vi "DTACQ - Read Data Size per Sample.vi"(8 "error in":errorcluster, 11 "Address":string) -> (0 "error out":errorcluster, 2 "Data Size":T1)   [LabVIEW 2017, in "Communications Library.lvlib"]
doc: "Read the size of data, for each sample point, from the analog in module. (eg. 16 bit or 32 bit dats?)"
uses:
  Communications Library.lvlib
  Typedefs/Data Size--Enum.ctl
  Typedefs/DTACQ Device Type--Enum.ctl
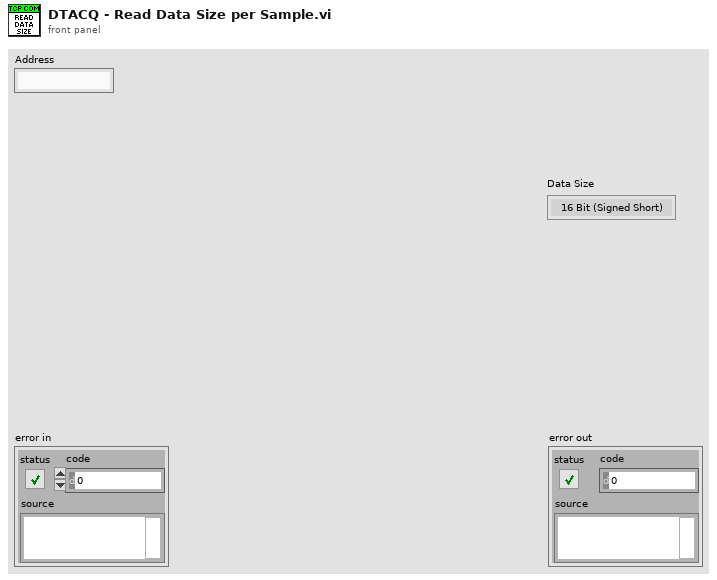
[diagram p1: front panel]
types:
  T1 = typedef "Communications Library.lvlib/Data Size--Enum.ctl" = enum16{"16 Bit (Signed Short)", "32 Bit (Signed Long)"}
  T2 = typedef "Communications Library.lvlib/DTACQ Device Type--Enum.ctl" = enum16{"Carrier", "Analog In Module", "Analog Out Module", "Generic Module"}
  T3 = typedef "Communications Library.lvlib/DTACQ Connection Data--Cluster.ctl" = cluster{"Description":string, "Address":string, "Port":u16, "timeout (ms)":i32, "Termination Character":string, "TCP Connection Reference":refnum<k5>, "Open Connection":bool}
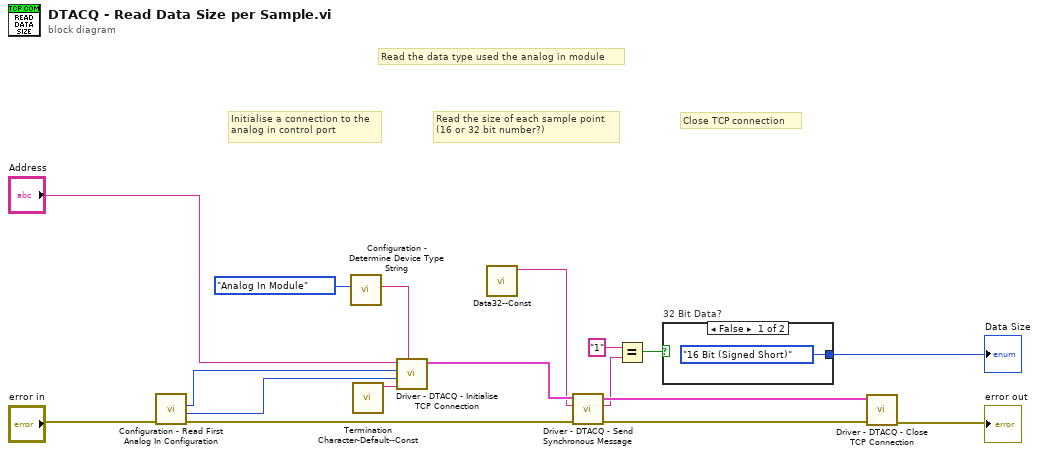
[diagram p0: block diagram]
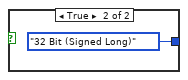
[diagram p2: hidden frame]
diagram:
  # "Initialise a connection to the\nanalog in control port"
  # "Read the data type used the analog in module"
  # "Close TCP connection"
  # "Read the size of each sample point\n(16 or 32 bit number?)"
  n1 = call "Configuration - Read First Analog In Configuration.vi"("error in"="error in") -> ("error out"=w12:errorcluster, "Timeout (ms)"=w1:i32, "Analog In Control Port"=w13:i32)  [unwired: 6 in, 2 out]
  n2 = call "Configuration - Determine Device Type String.vi"("Device Type In"=DTACQ_Device_Type--Enum."Analog In Module" ("Module Type")) -> ("Type String Out"=w14:string)  [unwired: 10 in]
  n3 = call "Termination Character-Default--Const.vi"() -> ("Termination Character"=w10:string)  [unwired: 11 in]
  n4 = call "Driver - DTACQ - Initialise TCP Connection.vi"("Description"=w14, "Termination Character"=w10, "timeout (ms)"=w1, "Port"=w13, "Address"="Address") -> ("DTACQ Connection Data Out"=w9:T3)  [unwired: 6 in]
  n5 = call "Data32--Const.vi"() -> ("Data32 Command"=w8:string)  [unwired: 11 in]
  n6 = call "Driver - DTACQ - Send Synchronous Message.vi"("error in"=w12, "Message to Send"=w8, "DTACQ Connection Data In"=w9) -> ("error out"=w7:errorcluster, "Read String"=w5:string, "DTACQ Connection Data Out"=w6:T3)  [unwired: 5 in, 1 out]
  n7 = Equal?(x="1", y=w5) -> (x = y?=w3:bool)
  n8 = case "32 Bit Data?" shown="False" w3 {
    tunnel: [Data_Size--Enum."16 Bit (Signed Short)" ("y") Data_Size--Enum."32 Bit (Signed Long)" ("y")] -> w2
    frame False {
    }
    frame True {
    }
  }
  "Data Size" <- w2
  n9 = call "Driver - DTACQ - Close TCP Connection.vi"("error in"=w7, "DTACQ Connection Data In"=w6) -> ("error out"=→"error out":errorcluster)  [unwired: 8 in, 1 out]
